vi "Spd_quat (SubVI).vi"(11 "Rotation":T1) -> (3 "Array":dbl[](array[numeric]))   [LabVIEW 2017]
uses:
  <vilib>/Analysis/coordinate.llb/Euler Rotation Order.ctl
  <vilib>/Analysis/NI_AALPro.lvlib
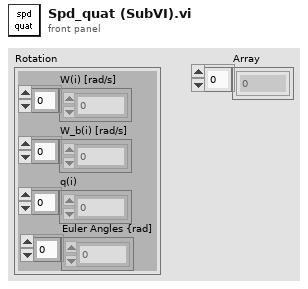
[diagram p1: front panel]
types:
  T1 = cluster{"W(i) [rad/s]":dbl[], "W_b(i) [rad/s]":dbl[], "q(i)":dbl[], "Euler Angles {rad]":dbl[]}
  T2 = typedef "NI_AALPro.lvlib/Euler Rotation Order.ctl" = u16
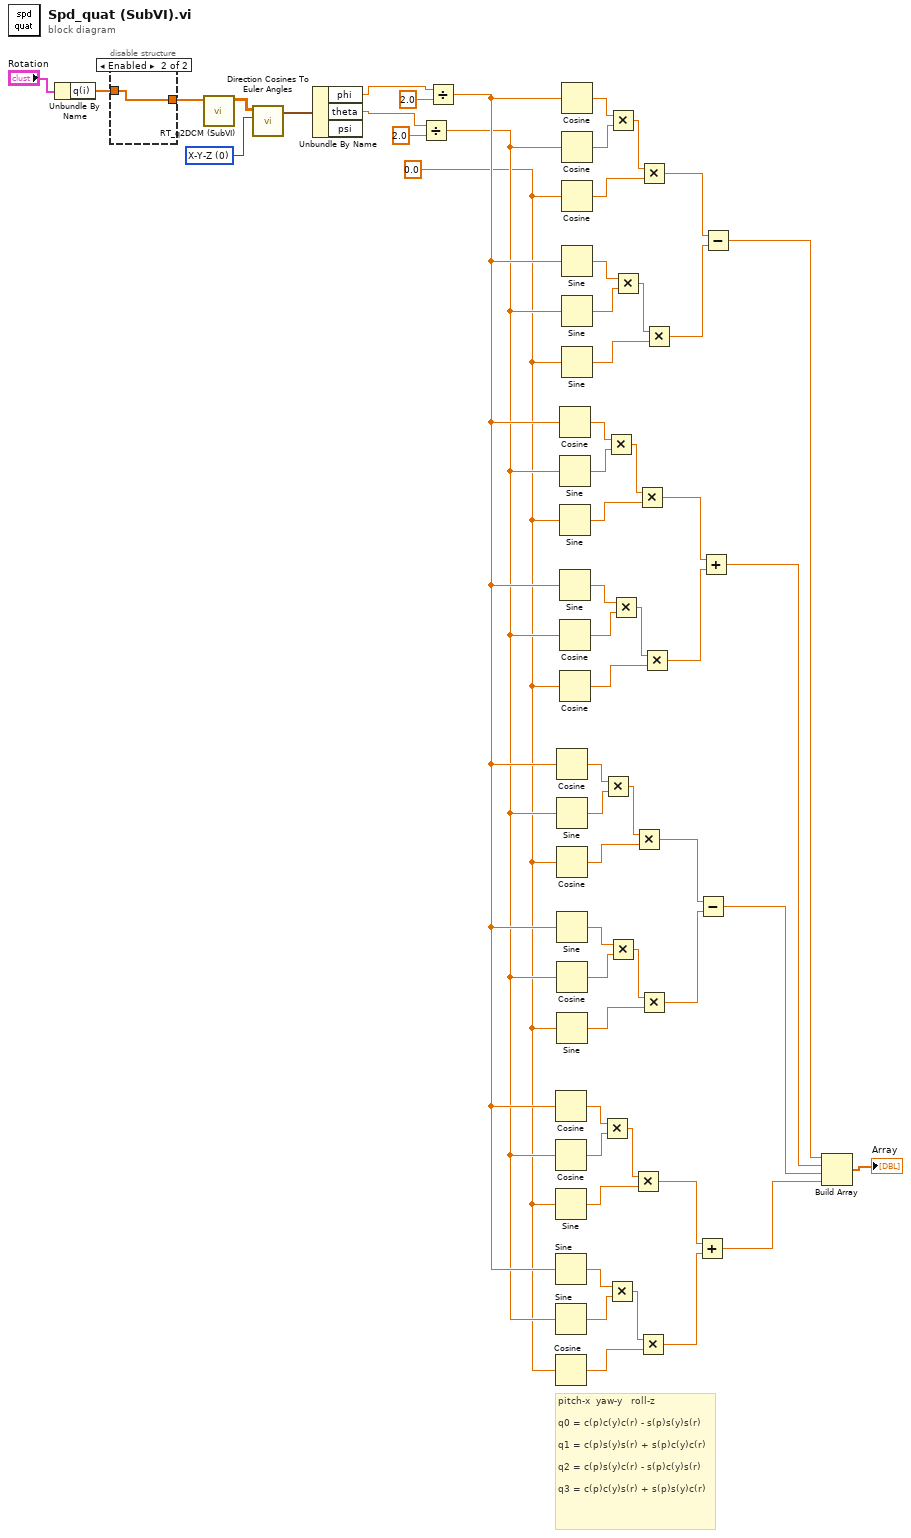
[diagram p0: block diagram]
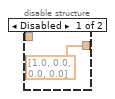
[diagram p2: hidden frame]
diagram:
  w45 = 0.0 ("x")
  w3 = T2 0 items=["X-Y-Z", "X-Z-Y", "Y-X-Z", "Y-Z-X", "Z-X-Y", "Z-Y-X", "X-Y-X", "X-Z-X", "Y-X-Y", "Y-Z-Y", "Z-X-Z", "Z-Y-Z"] ("rotation order")
  # "pitch-x  yaw-y   roll-z\n\nq0 = c(p)c(y)c(r) - s(p)s(y)s(r)\n\nq1 = c(p)s(y)s(r) + s(p)c(y)c(r)\n\nq2 = c(p)s(y)c(r) - s(p)c(y)s(r)\n\nq3 = c(p)c(y)s(r) + s(p)s(y)c(r)"
  n1 = Unbundle By Name("Rotation") -> ("q(i)"=w57:dbl[])
  n2 = disable-structure shown="Enabled" {
    disable-tunnel: w57 -> [_ w60]
    disable-tunnel: [dbl[] [1.0, 0.0, 0.0, 0.0] ("q(i)") w60] -> w1
    frame Disabled {
    }
    frame Enabled {
    }
  }
  n3 = call "RT_q2DCM (SubVI).vi"("Quaternion"=w1) -> ("DCM"=w4:dbl[][])  [unwired: 10 in]
  n4 = call <vilib>:"Direction Cosines To Euler Angles.vi"("rotation order"=w3, "Direction Cosines"=w4) -> ("Euler Angles"=w2:cluster{"phi":dbl, "theta":dbl, "psi":dbl})  [unwired: 8 in, 1 out]
  n5 = Unbundle By Name(w2) -> ("phi"=w53:dbl, "theta"=w54:dbl)  [unwired: 1 out]
  n6 = Divide(x=w54, y=2.0) -> (x/y=w55:dbl)
  n7 = Divide(x=w53, y=2.0) -> (x/y=w56:dbl)
  n8 = Cosine(x=w56) -> (cos(x)=w44:dbl)
  n9 = Cosine(x=w55) -> (cos(x)=w43:dbl)
  n10 = Sine(x=w45) -> (sin(x)=w41:dbl)
  n11 = Sine(x=w56) -> (sin(x)=w39:dbl)
  n12 = Sine(x=w55) -> (sin(x)=w38:dbl)
  n13 = Cosine(x=w45) -> (cos(x)=w37:dbl)
  n14 = Cosine(x=w56) -> (cos(x)=w25:dbl)
  n15 = Sine(x=w55) -> (sin(x)=w26:dbl)
  n16 = Cosine(x=w45) -> (cos(x)=w28:dbl)
  n17 = Sine(x=w56) -> (sin(x)=w30:dbl)
  n18 = Cosine(x=w55) -> (cos(x)=w31:dbl)
  n19 = Sine(x=w45) -> (sin(x)=w32:dbl)
  n20 = Cosine(x=w56) -> (cos(x)=w24:dbl)
  n21 = Sine(x=w55) -> (sin(x)=w23:dbl)
  n22 = Sine(x=w45) -> (sin(x)=w21:dbl)
  n23 = Sine(x=w56) -> (sin(x)=w19:dbl)
  n24 = Cosine(x=w55) -> (cos(x)=w18:dbl)
  n25 = Cosine(x=w45) -> (cos(x)=w17:dbl)
  n26 = Cosine(x=w56) -> (cos(x)=w5:dbl)
  n27 = Cosine(x=w55) -> (cos(x)=w6:dbl)
  n28 = Cosine(x=w45) -> (cos(x)=w8:dbl)
  n29 = Sine(x=w56) -> (sin(x)=w10:dbl)
  n30 = Sine(x=w55) -> (sin(x)=w11:dbl)
  n31 = Sine(x=w45) -> (sin(x)=w12:dbl)
  n32 = Multiply(x=w44, y=w43) -> (x*y=w42:dbl)
  n33 = Multiply(x=w25, y=w26) -> (x*y=w27:dbl)
  n34 = Multiply(x=w24, y=w23) -> (x*y=w22:dbl)
  n35 = Multiply(x=w39, y=w38) -> (x*y=w40:dbl)
  n36 = Multiply(x=w5, y=w6) -> (x*y=w7:dbl)
  n37 = Multiply(x=w30, y=w31) -> (x*y=w29:dbl)
  n38 = Multiply(x=w19, y=w18) -> (x*y=w20:dbl)
  n39 = Multiply(x=w10, y=w11) -> (x*y=w9:dbl)
  n40 = Multiply(x=w42, y=w41) -> (x*y=w36:dbl)
  n41 = Multiply(x=w27, y=w28) -> (x*y=w33:dbl)
  n42 = Multiply(x=w22, y=w21) -> (x*y=w16:dbl)
  n43 = Multiply(x=w40, y=w37) -> (x*y=w35:dbl)
  n44 = Multiply(x=w7, y=w8) -> (x*y=w13:dbl)
  n45 = Multiply(x=w29, y=w32) -> (x*y=w34:dbl)
  n46 = Multiply(x=w20, y=w17) -> (x*y=w15:dbl)
  n47 = Multiply(x=w9, y=w12) -> (x*y=w14:dbl)
  n48 = Add(x=w36, y=w35) -> (x+y=w49:dbl)
  n49 = Subtract(x=w33, y=w34) -> (x-y=w48:dbl)
  n50 = Add(x=w16, y=w15) -> (x+y=w47:dbl)
  n51 = Subtract(x=w13, y=w14) -> (x-y=w46:dbl)
  n52 = Build Array(w46, w47, w48, w49) -> (→"Array":dbl[])
